vi "GetItem.vi"(8 "Error In":errorcluster, 9 "Properties":T1[](array[typedef]), 10 "Player ID":i32, 11 "XBMC Ref":T2) -> (0 "Error Out":errorcluster, 1 "Response":string, 3 "XBMC Ref":T2)   [LabVIEW 2013, in "LMH-Kodi.lvlib" / "Player.lvlib"]
uses:
  Player.lvlib
  Private/Type Defs/XBMC Ref.ctl
  <vilib>/httpClient/ClientHandle.ctl
  Private/Type Defs/JSON_Objects/List_Fields_All.ctl
  Private/Type Defs/JSON_Objects/Player_GetItem.ctl
  Private/Type Defs/ID FGV State.ctl
  LMH-Kodi.lvlib
  <vilib>/httpClient/LabVIEWHTTPClient.lvlib
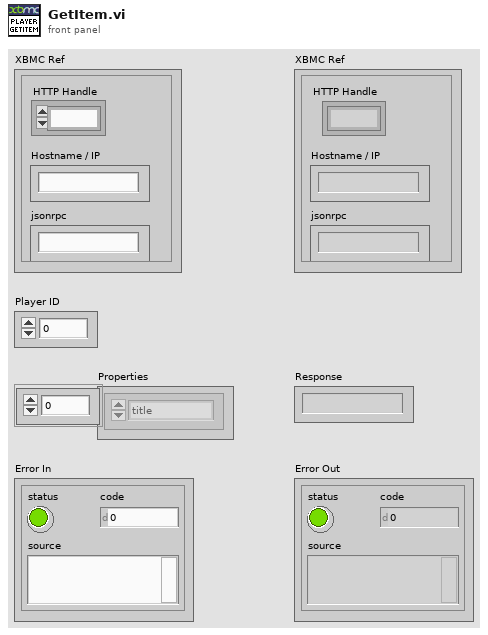
[diagram p1: front panel]
types:
  T1 = typedef "LMH-Kodi.lvlib/List_Fields_All.ctl" = enum16{"title", "artist", "albumartist", "genre", "year", "rating", "album", "track", "duration", "comment", "lyrics", "musicbrainztrackid", "musicbrainzartistid", "musicbrainzalbumid", "musicbrainzalbumartistid", "playcount", "fanart", "director", "trailer", "tagline", "plot", "plotoutline", "originaltitle", "lastplayed", "writer", "studio", "mpaa", "cast", "country", "imdbnumber", "premiered", "productioncode", "runtime", "set", "showlink", "streamdetails", "top250", "votes", "firstaired", "season", "episode", "showtitle", "thumbnail", "file", "resume", "artistid", "albumid", "tvshowid", "setid", "watchedepisodes", "disc", "tag", "art", "genreid", "displayartist", "albumartistid", "description", "theme", "mood", "style", "albumlabel", "sorttitle", "episodeguide", "uniqueid", "dateadded", "channel", "channeltype", "hidden", "locked", "channelnumber", "starttime", "endtime"}
  T2 = typedef "LMH-Kodi.lvlib/XBMC Ref.ctl" = cluster{"HTTP Handle":T3, "Hostname / IP":string, "jsonrpc":string}
  T3 = typedef "LabVIEWHTTPClient.lvlib/ClientHandle.ctl" = refnum<k1>
  T4 = enum16{"Player.GetActivePlayers", "Player.GetItem", "Player.GetProperties", "Player.GoTo", "Player.Move", "Player.Open", "Player.PlayPause", "Player.Rotate", "Player.Seek", "Player.SetAudioStream", "Player.SetPartyMode", "Player.SetRepeat", "Player.SetShuffle", "Player.SetSpeed", "Player.SetSubtitle", "Player.Stop", "Player.Zoom"}
  T5 = typedef "LMH-Kodi.lvlib/ID FGV State.ctl" = enum16{"Init", "Peek", "Get++"}
  T6 = typedef "LMH-Kodi.lvlib/Player_GetItem.ctl" = cluster{"method":string, "jsonrpc":string, "id":i32, "params":cluster{"playerid":i32, "properties":string[]}}
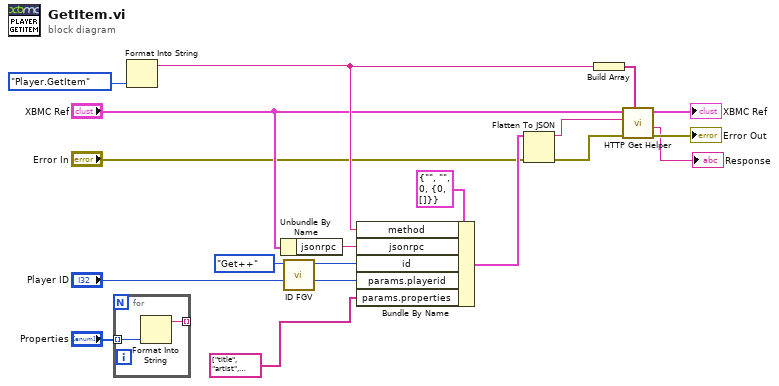
[diagram p0: block diagram]
diagram:
  n1 = for {
    tunnel: "Properties" -> [w20] mode=indexing
    tunnel: [w19] -> _ mode=indexing
    n2 = Format Into String(w20) -> (resulting string=w19:string)  [unwired: 3 in, 1 out]
  }
  n3 = Format Into String(T4."Player.GetItem" ("Method")) -> (resulting string=w12:string)  [unwired: 3 in, 1 out]
  n4 = Unbundle By Name("XBMC Ref") -> ("jsonrpc"=w4:string)
  n5 = call "ID FGV.vi"("FGV State"=ID_FGV_State."Get++") -> ("Value"=w5:i32)  [unwired: 10 in]
  n6 = Bundle By Name(cluster=T6 {"method"="", "jsonrpc"="", "id"=0, "params"={"playerid"=0, "properties"=[]}} ("Player.GetItem"), "method"=w12, "jsonrpc"=w4, "id"=w5, "params.playerid"="Player ID", "params.properties"=string[] ["title", "artist", "albumartist", "genre", "year", "rating", "album", "track", "duration", "comment", "lyrics", "musicbrainztrackid", "musicbrainzartistid", "musicbrainzalbumid", "musicbrainzalbumartistid", "playcount", "fanart", "director", "trailer", "tagline", "plot", "plotoutline", "originaltitle", "lastplayed", "writer", "studio", "mpaa", "cast", "country", "imdbnumber", "premiered", "productioncode", "runtime", "set", "showlink", "streamdetails", "top250", "votes", "firstaired", "season", "episode", "showtitle", "thumbnail", "file", "resume", "artistid", "albumid", "tvshowid", "setid", "watchedepisodes", "disc", "tag", "art", "genreid", "displayartist", "albumartistid", "description", "theme", "mood", "style", "albumlabel", "sorttitle", "episodeguide", "uniqueid", "dateadded", "channel", "channeltype", "hidden", "locked", "channelnumber", "starttime", "endtime"]) -> (w9:T6)
  n7 = Flatten To JSON(anything=w9, error in (no error)="Error In") -> (JSON string=w8:string, 11:w7:errorcluster)  [unwired: 1 in]
  n8 = Build Array(w12) -> (w15:string[])
  n9 = call "HTTP Get Helper.vi"("Error Arguments"=w15, "Error In"=w7, "JSON Request"=w8, "XBMC Ref"="XBMC Ref") -> ("Error Out"=→"Error Out":errorcluster, "Response"=→"Response":string, "XBMC Ref"=→"XBMC Ref":T2)  [unwired: 5 in]
